vi "Get Path Values.vi"(7 "Target (Process)":T1 items=["Process", "User", "Machine"], 8 "Error In":errorcluster) -> (0 "Error Out":errorcluster, 3 "Values[]":string[](array[string]))   [LabVIEW 2019, in "SLL Environment Variable.lvlib"]
doc: "Retrieve the <B>Values[]</B> stored in the path environment variable for the target environment."
uses:
  SLL Environment Variable.lvlib
  _Typedef/Target Environment Enum.ctl
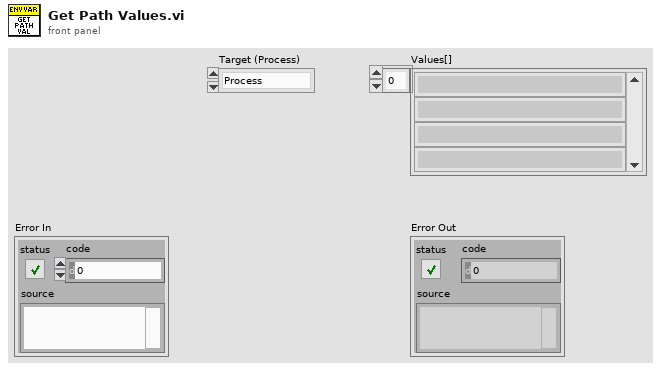
[diagram p1: front panel]
types:
  T1 = typedef "SLL Environment Variable.lvlib/Target Environment Enum.ctl" = i32
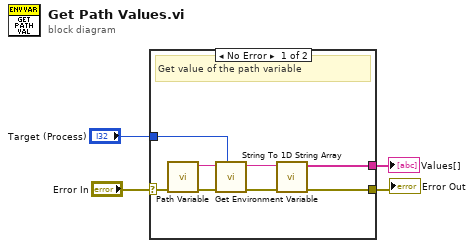
[diagram p0: block diagram]
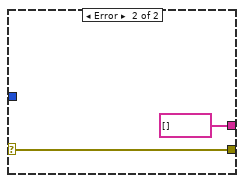
[diagram p2: hidden frame]
diagram:
  n1 = case shown="No Error" "Error In" {
    selector: "Error In" -> [w10 w11]
    tunnel: [w9 w11] -> w4
    tunnel: [w7 string[] []] -> w3
    tunnel: "Target (Process)" -> [w6 _]
    frame No Error {
      # "Get value of the path variable"
      n2 = call "Path Variable.vi"() -> ("Path Variable"=w5:string)  [unwired: 11 in]
      n3 = call "Get Environment Variable.vi"("Target (Process)"=w6, "Error In"=w10, "Name"=w5) -> ("Error Out"=w9:errorcluster, "Value"=w8:string)  [unwired: 7 in]
      n4 = call "String To 1D String Array.vi"("String"=w8) -> ("Array[]"=w7:string[])  [unwired: 10 in]
    }
    frame Error {
    }
  }
  "Error Out" <- w4
  "Values[]" <- w3
